vi "KI6221.vi"() -> ()   [LabVIEW 2019] (continued)
                            w597 = u16 2 ("f")
                            n439 = Equal?(x=w597, y=w598) -> (x = y?=w599:bool)
                            n440 = Select(t=w601, s=w599, f=w597) -> (s? t:f=w600:u16)
                            n441 = case shown="2" w600 {
                              tunnel: [FALSE ("VALID SETUP") TRUE ("VALID SETUP")] -> w605
                              tunnel: [TRUE ("VALID SETUP") FALSE ("VALID SETUP")] -> w604
                              frame 1, Default {
                              }
                              frame 2 {
                              }
                            }
                          }
                          frame 4 {
                            n442 = property on="GPIB 6220 label" class="Str"() -> ("Visible"=w637:bool)  [unwired: 2 in, 2 out]
                            n443 = case shown="True" w637 {
                              frame False {
                              }
                              frame True {
                                n444 = local write "Select the interface for the 6220/6221:"(2 ("Numeric 2")) -> ()
                              }
                            }
                            n445 = case shown="2, Default" w642 {
                              tunnel: [FALSE ("VALID SETUP") TRUE ("VALID SETUP")] -> w641
                              tunnel: [TRUE ("VALID SETUP") FALSE ("VALID SETUP")] -> w640
                              frame 1 {
                              }
                              frame 2, Default {
                              }
                            }
                          }
                          frame 5 {
                            n446 = local read "Verify instruments"() -> (w673:bool)
                            n447 = case shown="True" w673 {
                              tunnel: [0 2] -> w675
                              frame False {
                              }
                              frame True {
                              }
                            }
                            n448 = case shown="2, Default" w677 {
                              tunnel: [FALSE ("VALID SETUP") TRUE ("VALID SETUP")] -> w678
                              tunnel: [TRUE ("VALID SETUP") FALSE ("VALID SETUP")] -> w676
                              frame 1 {
                              }
                              frame 2, Default {
                              }
                            }
                          }
                          frame 6 {
                            n449 = local read "6220 Connect"() -> (w712:u16)
                            n450 = Equal To 0?(x=w712) -> (x = 0?=w715:bool)
                            n451 = Select(t=i16 2, s=w715, f=0 ("Numeric 2")) -> (s? t:f=w711:i32)
                            n452 = case shown="2, Default" w718 {
                              tunnel: [FALSE ("VALID SETUP") TRUE ("VALID SETUP")] -> w717
                              tunnel: [TRUE ("VALID SETUP") FALSE ("VALID SETUP")] -> w716
                              frame 1 {
                              }
                              frame 2, Default {
                              }
                            }
                          }
                          frame 7 {
                            n453 = case shown="8" w745 {
                              tunnel: [FALSE ("VALID SETUP") TRUE ("VALID SETUP")] -> w744
                              frame 0, Default {
                              }
                              frame 8 {
                              }
                            }
                            n454 = case shown="2, Default" w753 {
                              tunnel: [FALSE ("VALID SETUP") TRUE ("VALID SETUP")] -> w752
                              tunnel: [TRUE ("VALID SETUP") FALSE ("VALID SETUP")] -> w751
                              frame 1 {
                              }
                              frame 2, Default {
                              }
                            }
                          }
                          frame 8 {
                            n455 = case shown="1, 2, Default" w782 {
                              tunnel: [FALSE ("VALID SETUP") TRUE ("VALID SETUP")] -> w783
                              frame 3 {
                              }
                              frame 1, 2, Default {
                              }
                            }
                            n456 = case shown="9" w781 {
                              tunnel: [FALSE ("VALID SETUP") TRUE ("VALID SETUP")] -> w786
                              frame 0, Default {
                              }
                              frame 9 {
                              }
                            }
                            n457 = case shown="2, Default" w791 {
                              tunnel: [FALSE ("VALID SETUP") TRUE ("VALID SETUP")] -> w790
                              tunnel: [TRUE ("VALID SETUP") FALSE ("VALID SETUP")] -> w789
                              frame 1 {
                              }
                              frame 2, Default {
                              }
                            }
                          }
                          frame 9 {
                            n458 = case shown="2, Default" w829 {
                              tunnel: [FALSE ("VALID SETUP") TRUE ("VALID SETUP")] -> w828
                              tunnel: [TRUE ("VALID SETUP") FALSE ("VALID SETUP")] -> w827
                              frame 1 {
                              }
                              frame 2, Default {
                              }
                            }
                          }
                        }
                        n459 = property on="Select the current source model number:" class="Ring (strict)"("Visible"=w425, "Disabled"=w445) -> ()  [unwired: 2 in, 2 out]
                        n460 = property on="Select Network Card number:\n(default to zero)" class="DigNum (strict)"("Visible"=w439, "Disabled"=w438) -> ()  [unwired: 2 in, 2 out]
                        n461 = property on="Select the interface for the 6220/6221:" class="Ring (strict)"("Visible"=w442, "Disabled"=w441) -> ()  [unwired: 2 in, 2 out]
                        n462 = property on="Select GPIB Board number:\n(default to zero)" class="DigNum (strict)"("Visible"=w417, "Disabled"=w436) -> ()  [unwired: 2 in, 2 out]
                        n463 = property on="CANCEL" class="Bool"("Visible"=w420) -> ()  [unwired: 2 in, 2 out]
                        n464 = property on="Select the nanovoltmeter model number:" class="Ring (strict)"("Visible"=w444, "Disabled"=w443) -> ()  [unwired: 2 in, 2 out]
                        n465 = property on="Power:" class="Ring (strict)"("Visible"=w418, "Disabled"=w437) -> ()  [unwired: 2 in, 2 out]
                        n466 = property on="Select GPIB Address number \nof the current source:" class="DigNum (strict)"("Visible"=w416, "Disabled"=w440) -> ()  [unwired: 2 in, 2 out]
                        n467 = property on="NEXT" class="Bool"("Disabled"=w398) -> ()  [unwired: 2 in, 2 out]
                        n468 = Equal To 0?(x=w398) -> (x = 0?=w396:bool)
                        n469 = Not(x=w394) -> (.not. x?=w395:bool)
                        n470 = And(x=w396, y=w395) -> (x .and. y?=w397:bool)
                        n471 = case shown="True" w397 {
                          frame False {
                          }
                          frame True {
                            n472 = property on="NEXT" class="Bool"("Key Focus"=TRUE) -> ()  [unwired: 2 in, 2 out]
                          }
                        }
                        n473 = property on="instrument status" class="Str"("Visible"=w418) -> ()  [unwired: 2 in, 2 out]
                        n474 = property on="Input instrument IP Address:" class="DigNum (strict)"("Visible"=w435, "Disabled"=w434) -> ()  [unwired: 2 in, 2 out]
                        n475 = property on=".  IP#3" class="DigNum (strict)"("Visible"=w431, "Disabled"=w430) -> ()  [unwired: 2 in, 2 out]
                        n476 = property on=".  IP#2" class="DigNum (strict)"("Visible"=w433, "Disabled"=w432) -> ()  [unwired: 2 in, 2 out]
                        n477 = property on=".  IP#4" class="DigNum (strict)"("Visible"=w429, "Disabled"=w428) -> ()  [unwired: 2 in, 2 out]
                        n478 = property on="LOW to EARTH 2" class="Ring (strict)"("Visible"=w403, "Disabled"=w413) -> ()  [unwired: 2 in, 2 out]
                        n479 = property on="6220 Connect" class="Ring (strict)"("Visible"=w422, "Disabled"=w426) -> ()  [unwired: 2 in, 2 out]
                        n480 = property on="HI IMP devices?" class="Ring (strict)"("Visible"=w423, "Disabled"=w427) -> ()  [unwired: 2 in, 2 out]
                        n481 = case shown="True" w394 {
                          frame False {
                          }
                          frame True {
                            n482 = property on="OK" class="Bool (strict)"("Key Focus"=TRUE) -> ()  [unwired: 2 in, 2 out]
                          }
                        }
                        n483 = case shown="3" w401 {
                          tunnel: [TRUE FALSE] -> w400
                          frame 3 {
                          }
                          frame 1, 2, Default {
                          }
                        }
                        n484 = And(x=w400, y=w403) -> (x .and. y?=w402:bool)
                        n485 = property on="OK" class="Bool (strict)"("Visible"=w394) -> ()  [unwired: 2 in, 2 out]
                        n486 = property on="CAP IN" class="Ring (strict)"("Visible"=w402, "Disabled"=w404) -> ()  [unwired: 2 in, 2 out]
                        n487 = case shown="True" w407 {
                          tunnel: w412 -> [_ w462]
                          tunnel: w401 -> [_ w461]
                          tunnel: w411 -> [_ w460]
                          tunnel: w410 -> [_ w459]
                          tunnel: w409 -> [_ w458]
                          tunnel: w408 -> [_ w457]
                          tunnel: w406 -> [_ w451]
                          frame False {
                          }
                          frame True {
                            n488 = call "DecideWindow.vi"("Default Path"=w462, "NanoVoltmeter"=w461, "INDEX"=w451, "SOURCE 4"=w460, "MEASURE 4"=w458, "FLOAT 4"=w457, "CAP OUT 4"=w459, "wizard?"=1) -> ("SOURCE"=w455:i32, "MEASURE"=w454:i32, "FLOAT"=w453:i32, "CAP OUT"=w452:i32, "INDEX OUT"=w450:i32)  [unwired: 3 in]
                            n489 = local write "NEXT FLAG"(w450) -> ()
                            n490 = local write "LOW to EARTH 2"(w453) -> ()
                            n491 = local write "HI IMP devices?"(w454) -> ()
                            n492 = local write "6220 Connect"(w455) -> ()
                            n493 = local write "CAP IN"(w452) -> ()
                          }
                        }
                        n494 = property on="Main intro bar" class="Pict"("Visible"=w422) -> ()  [unwired: 2 in, 2 out]
                        n495 = property on="DUT connect HELP" class="Bool"("Visible"=w405) -> ()  [unwired: 2 in, 2 out]
                        n496 = property on="Src Connect HELP" class="Bool"("Visible"=w405) -> ()  [unwired: 2 in, 2 out]
                        n497 = property on="Lo earth HELP" class="Bool"("Visible"=w405) -> ()  [unwired: 2 in, 2 out]
                        n498 = property on="nVm C HELP" class="Bool"("Visible"=w405) -> ()  [unwired: 2 in, 2 out]
                      }
                    }
                  }
                  frame 1 {
                    w877 = TRUE ("Visible")
                    w885 = u8 0 ("Disabled")
                    # "PRESENT"
                    n499 = property on="Src Connect HELP" class="Bool"("Visible"=w877) -> ()  [unwired: 2 in, 2 out]
                    n500 = Equal?(x="Select the current source model number:", y=u16 2) -> (x = y?=w883:bool)
                    n501 = property on="DUT connect HELP" class="Bool"("Visible"=w877) -> ()  [unwired: 2 in, 2 out]
                    n502 = Not(x=w883) -> (.not. x?=w879:bool)
                    n503 = property on="Select the interface for the 6220/6221:" class="Ring (strict)"("Visible"=w883) -> ()  [unwired: 2 in, 2 out]
                    n504 = property on="GPIB 6220 label" class="Str"("Visible"=w879) -> ()  [unwired: 2 in, 2 out]
                    n505 = Equal?(x="Select the current source model number:", y=u16 1) -> (x = y?=w872:bool)
                    n506 = Select(t=u16 2, s=w872, f="Select the interface for the 6220/6221:") -> (s? t:f=w870:u16)
                    n507 = property on="Lo earth HELP" class="Bool"("Visible"=w877) -> ()  [unwired: 2 in, 2 out]
                    n508 = Equal?(x=w870, y=u16 2) -> (x = y?=w881:bool)
                    n509 = local write "Select the interface for the 6220/6221:"(w870) -> ()
                    n510 = Or(x=w881, y=w879) -> (x .or. y?=w878:bool)
                    n511 = Not(x=w878) -> (.not. x?=w880:bool)
                    n512 = property on="Select GPIB Address number \nof the current source:" class="DigNum (strict)"("Visible"=w878, "Disabled"=w885) -> ()  [unwired: 2 in, 2 out]
                    n513 = property on="Select GPIB Board number:\n(default to zero)" class="DigNum (strict)"("Visible"=w878, "Disabled"=w885) -> ()  [unwired: 2 in, 2 out]
                    n514 = property on=".  IP#4" class="DigNum (strict)"("Visible"=w880, "Disabled"=w885) -> ()  [unwired: 2 in, 2 out]
                    n515 = property on="Select Network Card number:\n(default to zero)" class="DigNum (strict)"("Visible"=w880, "Disabled"=w885) -> ()  [unwired: 2 in, 2 out]
                    n516 = property on="Input instrument IP Address:" class="DigNum (strict)"("Visible"=w880, "Disabled"=w885) -> ()  [unwired: 2 in, 2 out]
                    n517 = property on=".  IP#2" class="DigNum (strict)"("Visible"=w880, "Disabled"=w885) -> ()  [unwired: 2 in, 2 out]
                    n518 = property on=".  IP#3" class="DigNum (strict)"("Visible"=w880, "Disabled"=w885) -> ()  [unwired: 2 in, 2 out]
                    n519 = case shown="1, 2, Default" w876 {
                      tunnel: [TRUE FALSE] -> w875
                      frame 3 {
                      }
                      frame 1, 2, Default {
                      }
                    }
                    n520 = property on="CAP IN" class="Ring (strict)"("Visible"=w875) -> ()  [unwired: 2 in, 2 out]
                    n521 = property on="nVm C HELP" class="Bool"("Visible"=w875) -> ()  [unwired: 2 in, 2 out]
                  }
                }
                n522 = case shown="True" "nVm C HELP" {
                  tunnel: w293 -> [_ w373]
                  tunnel: "HI IMP devices?" -> [_ w372]
                  tunnel: w292 -> [_ w370]
                  tunnel: w298 -> [_ w369]
                  tunnel: "LOW to EARTH 2" -> [_ w368]
                  tunnel: "CAP IN" -> [_ w363]
                  frame False {
                  }
                  frame True {
                    n523 = call "DecideWindow.vi"("Default Path"=w369, "NanoVoltmeter"=w370, "INDEX"=3, "SOURCE 4"=w373, "MEASURE 4"=w372, "FLOAT 4"=w368, "CAP OUT 4"=w363, "wizard?"=0) -> ("SOURCE"=w367:i32, "MEASURE"=w366:i32, "FLOAT"=w365:i32, "CAP OUT"=w364:i32)  [unwired: 3 in, 1 out]
                    n524 = local write "LOW to EARTH 2"(w365) -> ()
                    n525 = local write "6220 Connect"(w367) -> ()
                    n526 = local write "HI IMP devices?"(w366) -> ()
                    n527 = local write "CAP IN"(w364) -> ()
                  }
                }
                n528 = case shown="True" "Src Connect HELP" {
                  tunnel: "CAP IN" -> [_ w360]
                  tunnel: "LOW to EARTH 2" -> [_ w359]
                  tunnel: w292 -> [_ w358]
                  tunnel: "HI IMP devices?" -> [_ w357]
                  tunnel: w293 -> [_ w356]
                  tunnel: w298 -> [_ w355]
                  frame False {
                  }
                  frame True {
                    n529 = call "DecideWindow.vi"("Default Path"=w355, "NanoVoltmeter"=w358, "INDEX"=0, "SOURCE 4"=w356, "MEASURE 4"=w357, "FLOAT 4"=w359, "CAP OUT 4"=w360, "wizard?"=0) -> ("SOURCE"=w353:i32, "MEASURE"=w352:i32, "FLOAT"=w351:i32, "CAP OUT"=w354:i32)  [unwired: 3 in, 1 out]
                    n530 = local write "LOW to EARTH 2"(w351) -> ()
                    n531 = local write "HI IMP devices?"(w352) -> ()
                    n532 = local write "6220 Connect"(w353) -> ()
                    n533 = local write "CAP IN"(w354) -> ()
                  }
                }
                n534 = case shown="True" "DUT connect HELP" {
                  tunnel: "CAP IN" -> [_ w348]
                  tunnel: "LOW to EARTH 2" -> [_ w347]
                  tunnel: w292 -> [_ w346]
                  tunnel: "HI IMP devices?" -> [_ w345]
                  tunnel: w293 -> [_ w344]
                  tunnel: w298 -> [_ w343]
                  frame False {
                  }
                  frame True {
                    n535 = call "DecideWindow.vi"("Default Path"=w343, "NanoVoltmeter"=w346, "INDEX"=1, "SOURCE 4"=w344, "MEASURE 4"=w345, "FLOAT 4"=w347, "CAP OUT 4"=w348, "wizard?"=0) -> ("SOURCE"=w342:i32, "MEASURE"=w341:i32, "FLOAT"=w340:i32, "CAP OUT"=w339:i32)  [unwired: 3 in, 1 out]
                    n536 = local write "LOW to EARTH 2"(w340) -> ()
                    n537 = local write "HI IMP devices?"(w341) -> ()
                    n538 = local write "6220 Connect"(w342) -> ()
                    n539 = local write "CAP IN"(w339) -> ()
                  }
                }
                n540 = case shown="True" "Lo earth HELP" {
                  tunnel: "CAP IN" -> [_ w336]
                  tunnel: "LOW to EARTH 2" -> [_ w335]
                  tunnel: w292 -> [_ w334]
                  tunnel: "HI IMP devices?" -> [_ w333]
                  tunnel: w293 -> [_ w332]
                  tunnel: w298 -> [_ w331]
                  frame False {
                  }
                  frame True {
                    n541 = call "DecideWindow.vi"("Default Path"=w331, "NanoVoltmeter"=w334, "INDEX"=2, "SOURCE 4"=w332, "MEASURE 4"=w333, "FLOAT 4"=w335, "CAP OUT 4"=w336, "wizard?"=0) -> ("SOURCE"=w327:i32, "MEASURE"=w328:i32, "FLOAT"=w329:i32, "CAP OUT"=w330:i32)  [unwired: 3 in, 1 out]
                    n542 = local write "LOW to EARTH 2"(w329) -> ()
                    n543 = local write "HI IMP devices?"(w328) -> ()
                    n544 = local write "6220 Connect"(w327) -> ()
                    n545 = local write "CAP IN"(w330) -> ()
                  }
                }
                n546 = case shown="True" "Case Constant\n(See Context Help) 3" {
                  tunnel: w292 -> [_ w323]
                  frame False {
                  }
                  frame True {
                    n547 = case shown="3" w323 {
                      tunnel: [TRUE FALSE] -> w324
                      frame 3 {
                      }
                      frame 1, 2, Default {
                      }
                    }
                    n548 = property on="nVm C HELP" class="Bool"("Visible"=w324) -> ()  [unwired: 2 in, 2 out]
                    n549 = property on="CAP IN" class="Ring (strict)"("Visible"=w324) -> ()  [unwired: 2 in, 2 out]
                  }
                }
                n550 = call "Measure Connect HELP"("Enable"=w303) -> ()  [unwired: 9 in, 2 out]
                n551 = call "Low to Earth HELP"("Enable"=w303) -> ()  [unwired: 9 in, 2 out]
                n552 = call "Source Connect HELP"("Enable"=w303) -> ()  [unwired: 9 in, 2 out]
              }
              frame "CONN GUIDE" {
                w1092 = u8 0 ("Disabled")
                # "How Do I Decide Links"
                # "BUTTONS INVISIBLE IN THIS VERSION OF THE PANEL."
                # "Global Buttons"
                # "PREVIOUS & START OVER BUTTON CONTROLS"
                # "GUIDE BUTTON CONTROLS"
                n553 = Not Equal?(x="4 step TABS", y="4 step TABS LAST") -> (x != y?=w1096:bool)
                n554 = case shown="True" "END OF GUIDE" {
                  frame False {
                  }
                  frame True {
                    n555 = local write "4 step TABS"(T3."step 4" ("4 step TABS")) -> ()
                  }
                }
                n556 = case shown="True" "start of guide" {
                  frame False {
                  }
                  frame True {
                    n557 = local write "4 step TABS"(T3."step 1" ("4 step TABS")) -> ()
                  }
                }
                n558 = case shown="True" "Previous" {
                  tunnel: "4 step TABS" -> [_ w1211]
                  frame False {
                  }
                  frame True {
                    n559 = Decrement(x=w1211) -> (x-1=w1210:T3)
                    n560 = local write "4 step TABS"(w1210) -> ()
                  }
                }
                n561 = property on="Main Tabs" class="TabCtl (strict)"("Page Selector Visible"=TRUE) -> ()  [unwired: 2 in, 2 out]
                n562 = case shown="True" "NEXT GUIDE" {
                  tunnel: "4 step TABS" -> [_ w1209]
                  frame False {
                  }
                  frame True {
                    n563 = Increment(x=w1209) -> (x+1=w1208:T3)
                    n564 = local write "4 step TABS"(w1208) -> ()
                  }
                }
                n565 = case shown="True" w1096 {
                  tunnel: "4 step TABS" -> [_ w1191]
                  frame False {
                  }
                  frame True {
                    n566 = case shown="\"step 4\"" w1191 {
                      tunnel: [u8 2 ("Disabled") w1198 u8 0 ("Disabled") w1203 w1205] -> w1193
                      tunnel: [u8 0 ("Disabled") w1198 u8 2 ("Disabled") w1203 w1205] -> w1192
                      tunnel: [FALSE FALSE TRUE FALSE FALSE] -> w1190
                      frame "step 1", Default {
                      }
                      frame "step 3" {
                        w1198 = u8 0 ("Disabled")
                      }
                      frame "step 4" {
                      }
                      frame "final" {
                        w1203 = u8 0 ("Disabled")
                      }
                      frame "step 2" {
                        w1205 = u8 0 ("Disabled")
                      }
                    }
                    n567 = local write "4 step TABS LAST"(w1191) -> ()
                    n568 = property on="start of guide" class="Bool"("Disabled"=w1193) -> ()  [unwired: 2 in, 2 out]
                    n569 = property on="Previous" class="Bool"("Disabled"=w1193) -> ()  [unwired: 2 in, 2 out]
                    n570 = property on="END OF GUIDE" class="Bool"("Disabled"=w1192) -> ()  [unwired: 2 in, 2 out]
                    n571 = property on="NEXT GUIDE" class="Bool"("Disabled"=w1192) -> ()  [unwired: 2 in, 2 out]
                    n572 = property on="Nearby AC voltages" class="Bool (strict)"("Visible"=w1190) -> ()  [unwired: 2 in, 2 out]
                    n573 = property on="AC HELP" class="Bool"("Visible"=w1190) -> ()  [unwired: 2 in, 2 out]
                    n574 = property on="HAZARD HELP" class="Bool"("Visible"=w1190) -> ()  [unwired: 2 in, 2 out]
                    n575 = property on="H,L,G Haz volt" class="Bool (strict)"("Visible"=w1190) -> ()  [unwired: 2 in, 2 out]
                  }
                }
                n576 = property on="EXIT 2" class="Bool (strict)"("Disabled"=w1092) -> ()  [unwired: 2 in, 2 out]
                n577 = property on="SAVE 2" class="Bool"("Disabled"=w1092) -> ()  [unwired: 2 in, 2 out]
                n578 = case shown="True" "setup wizard" {
                  frame False {
                  }
                  frame True {
                    n579 = case shown="True" "CONNECT\nONLY FLAG" {
                      tunnel: [T2."CONN CONFIG" ("COMM\nTab Control") T2."STARTUP" ("COMM\nTab Control")] -> w1214
                      frame False {
                      }
                      frame True {
                      }
                    }
                    n580 = property on="COMM\nTab Control" class="TabCtl (strict)"("Value"=w1214) -> ()  [unwired: 2 in, 2 out]
                  }
                }
                n581 = case shown="True" "RETURN TO SPLASH SCREEN" {
                  frame False {
                  }
                  frame True {
                    n582 = property on="COMM\nTab Control" class="TabCtl (strict)"("Value"=T2."STARTUP" ("COMM\nTab Control")) -> ()  [unwired: 2 in, 2 out]
                  }
                }
                n583 = Not Equal?(x="Nearby AC voltages", y="Nearby AC voltages LAST") -> (x != y?=w1087:bool)
                n584 = Not Equal?(x="H,L,G Haz volt", y="H,L,G Haz volt LAST") -> (x != y?=w1086:bool)
                n585 = Not Equal?(x="CAP", y="CAP LAST") -> (x != y?=w1085:bool)
                n586 = Not Equal?(x="COMM TAB LAST", y=w1093) -> (x != y?=w1081:bool)
                n587 = Compound Arithmetic op=OR(w1081, w1087, w1086, w1085) -> (w1088:bool)
                n588 = case shown="True" w1088 {
                  tunnel: w1093 -> [_ w1166]
                  tunnel: "Nearby AC voltages" -> [_ w1116]
                  tunnel: "H,L,G Haz volt" -> [_ w1114]
                  tunnel: "CAP" -> [_ w1117]
                  tunnel: w1081 -> [_ w1113]
                  frame False {
                  }
                  frame True {
                    w1122 = ".png" ("string")
                    w1129 = "Guide" ("string")
                    # "Initialize pictures when you get to the GUIDE GUI PANEL."
                    n589 = local read "6220 Connect"() -> (w1115:u16)
                    n590 = local read "Select the interface for the 6220/6221:"() -> (w1167:u16)
                    n591 = local write "COMM TAB LAST"(w1166) -> ()
                    n592 = Decrement(x=w1115) -> (x-1=w1139:u16)
                    n593 = Number To Decimal String(number=w1139) -> (decimal integer string=w1138:string)  [unwired: 1 in]
                    n594 = local read "LOW to EARTH 2"() -> (w1168:u16)
                    n595 = Number To Decimal String(number=w1168) -> (decimal integer string=w1118:string)  [unwired: 1 in]
                    n596 = local write "CAP LAST"(w1117) -> ()
                    n597 = local read "Default path"() -> (w1130:path)
                    n598 = local read "HI IMP devices?"() -> (w1121:u16)
                    n599 = Decrement(x=w1167) -> (x-1=w1163:u16)
                    n600 = Number To Decimal String(number=w1163) -> (decimal integer string=w1128:string)  [unwired: 1 in]
                    n601 = case shown="1" w1121 {
                      tunnel: [u16 1 ("HI IMP devices?") u16 0 ("HI IMP devices?")] -> w1120
                      frame 0, Default {
                      }
                      frame 1 {
                      }
                    }
                    n602 = Number To Decimal String(number=w1120) -> (decimal integer string=w1119:string)  [unwired: 1 in]
                    n603 = Boolean To (0,1)(Boolean=w1116) -> (0, 1=w1165:i16)
                    n604 = local write "Nearby AC voltages LAST"(w1116) -> ()
                    n605 = Number To Decimal String(number=w1165) -> (decimal integer string=w1157:string)  [unwired: 1 in]
                    n606 = Number To Decimal String(number=2 ("y")) -> (decimal integer string=w1143:string)  [unwired: 1 in]
                    n607 = Number To Decimal String(number=4 ("y")) -> (decimal integer string=w1159:string)  [unwired: 1 in]
                    n608 = Number To Decimal String(number=1 ("y")) -> (decimal integer string=w1134:string)  [unwired: 1 in]
                    n609 = Concatenate Strings(w1129, w1143, w1138, w1118, w1122) -> (w1144:string)
                    n610 = Concatenate Strings(w1129, w1134, w1128, w1122) -> (w1135:string)
                    n611 = Build Path(base path=w1130, name or relative path=w1144) -> (appended path=w1146:path)
                    n612 = Build Path(base path=w1130, name or relative path=w1135) -> (appended path=w1137:path)
                    n613 = call <vilib>:"Read PNG File.vi"("path to PNG file"=w1146) -> ("error out"=w1141:errorcluster, "image data"=w1145:T13)  [unwired: 8 in, 1 out]
                    n614 = Number To Decimal String(number=3 ("y")) -> (decimal integer string=w1150:string)  [unwired: 1 in]
                    n615 = Concatenate Strings(w1129, w1150, w1119, w1122) -> (w1151:string)
                    n616 = Build Path(base path=w1130, name or relative path=w1151) -> (appended path=w1153:path)
                    n617 = call <vilib>:"Read PNG File.vi"("path to PNG file"=w1137) -> ("error out"=w1132:errorcluster, "image data"=w1136:T13)  [unwired: 8 in, 1 out]
                    n618 = call <vilib>:"Read PNG File.vi"("path to PNG file"=w1153) -> ("error out"=w1148:errorcluster, "image data"=w1152:T13)  [unwired: 8 in, 1 out]
                    n619 = call <vilib>:"Draw Flattened Pixmap.vi"("image data"=w1145) -> ("new picture"=w1140:picture)  [unwired: 8 in]
                    n620 = case shown="2, Default" w1115 {
                      tunnel: [2 ("y") 0 ("y")] -> w1112
                      tunnel: [TRUE ("H,L,G Haz volt") w1174] -> w1111
                      tunnel: w1114 -> [_ w1174]
                      frame 2, Default {
                      }
                      frame 1 {
                      }
                    }
                    n621 = Boolean To (0,1)(Boolean=w1111) -> (0, 1=w1164:i16)
                    n622 = Number To Decimal String(number=w1164) -> (decimal integer string=w1156:string)  [unwired: 1 in]
                    n623 = Concatenate Strings(w1129, w1159, w1138, w1119, w1118, w1157, w1156, w1122) -> (w1160:string)
                    n624 = Build Path(base path=w1130, name or relative path=w1160) -> (appended path=w1162:path)
                    n625 = call <vilib>:"Read PNG File.vi"("path to PNG file"=w1162) -> ("error out"=w1155:errorcluster, "image data"=w1161:T13)  [unwired: 8 in, 1 out]
                    n626 = call <vilib>:"Draw Flattened Pixmap.vi"("image data"=w1161) -> ("new picture"=w1154:picture)  [unwired: 8 in]
                    n627 = case shown="No Error" w1155 {
                      tunnel: w1154 -> [w1188 _]
                      tunnel: [FALSE TRUE] -> w1126
                      frame No Error {
                        n628 = local write "step 4 pic"(w1188) -> ()
                      }
                      frame Error {
                      }
                    }
                    n629 = call <vilib>:"Draw Flattened Pixmap.vi"("image data"=w1136) -> ("new picture"=w1131:picture)  [unwired: 8 in]
                    n630 = call <vilib>:"Draw Flattened Pixmap.vi"("image data"=w1152) -> ("new picture"=w1147:picture)  [unwired: 8 in]
                    n631 = case shown="No Error" w1141 {
                      tunnel: w1140 -> [w1182 _]
                      tunnel: [FALSE TRUE] -> w1124
                      frame No Error {
                        n632 = local write "step 2 pic"(w1182) -> ()
                      }
                      frame Error {
                      }
                    }
                    n633 = case shown="No Error" w1132 {
                      tunnel: w1131 -> [w1179 _]
                      tunnel: [FALSE TRUE] -> w1123
                      frame No Error {
                        n634 = local write "step 1 pic"(w1179) -> ()
                      }
                      frame Error {
                      }
                    }
                    n635 = case shown="No Error" w1148 {
                      tunnel: w1147 -> [w1185 _]
                      tunnel: [FALSE TRUE] -> w1125
                      frame No Error {
                        n636 = local write "step 3 pic"(w1185) -> ()
                      }
                      frame Error {
                      }
                    }
                    n637 = property on="H,L,G Haz volt" class="Bool (strict)"("Value"=w1111, "Disabled"=w1112) -> ()  [unwired: 2 in, 2 out]
                    n638 = case shown="True" w1113 {
                      frame False {
                      }
                      frame True {
                        n639 = local write "4 step TABS"(T3."step 1" ("4 step TABS")) -> ()
                        n640 = property on="NEXT GUIDE" class="Bool"("Disabled"=u8 0) -> ()  [unwired: 2 in, 2 out]
                        n641 = property on="Previous" class="Bool"("Disabled"=u8 2) -> ()  [unwired: 2 in, 2 out]
                      }
                    }
                    n642 = local write "H,L,G Haz volt LAST"(w1111) -> ()
                    n643 = property on="HAZARD HELP" class="Bool"("Disabled"=w1112) -> ()  [unwired: 2 in, 2 out]
                    n644 = Compound Arithmetic op=OR(w1126, w1125, w1124, w1123) -> (w1127:bool)
                    n645 = call "Images not found"("Enable"=w1127) -> ()  [unwired: 9 in, 2 out]
                  }
                }
                n646 = local read "Default path"() -> (w1078:path)
                n647 = case shown="True" "HAZARD HELP" {
                  tunnel: w1078 -> [_ w1108]
                  frame False {
                  }
                  frame True {
                    n648 = call "DecideWindow.vi"("Default Path"=w1108, "INDEX"=5, "wizard?"=0) -> ()  [unwired: 8 in, 5 out]
                  }
                }
                n649 = case shown="True" "AC HELP" {
                  tunnel: w1078 -> [_ w1105]
                  frame False {
                  }
                  frame True {
                    n650 = call "DecideWindow.vi"("Default Path"=w1105, "INDEX"=6, "wizard?"=0) -> ()  [unwired: 8 in, 5 out]
                  }
                }
              }
              frame "STEP CONFIG" {
                w1218 = u8 2 ("Disabled")
                # "Step setup CANCEL. Returns all VARS to previous values."
                # "This vi updates the VARS for the step source. Used when OK is \nclicked."
                # "Controls/Indicators referenced, not used."
                # "This enables the OK button once a name is entered."
                # "Turns off TABS MUST HIT OK or CANCEL to CONTINUE."
                n651 = case shown="True" "step setup OK" {
                  frame False {
                  }
                  frame True {
                    n652 = control-ref of="STEP EDIT VAR"() -> (w1230:refnum<vi>)
                    n653 = control-ref of="GPIB Address:"() -> (w1238:refnum<vi>)
                    n654 = control-ref of="DELAY in mS"() -> (w1232:refnum<vi>)
                    n655 = control-ref of="GO TO LEVEL:                *NOTE - MUST include <LEVEL>"() -> (w1239:refnum<vi>)
                    n656 = control-ref of="INSTRUMENT NAME:"() -> (w1237:refnum<vi>)
                    n657 = control-ref of="VERIFY:"() -> (w1236:refnum<vi>)
                    n658 = control-ref of="RESPONSE STRING:"() -> (w1235:refnum<vi>)
                    n659 = control-ref of="CONFIGURE:"() -> (w1234:refnum<vi>)
                    n660 = control-ref of="DEACTIVATE:"() -> (w1233:refnum<vi>)
                    n661 = control-ref of="MASTER DRIVER Array"() -> (w1231:refnum<vi>)
                    n662 = control-ref of="Default path"() -> (w1241:refnum<vi>)
                    n663 = control-ref of="Select step source:"() -> (w1240:refnum<vi>)
                    n664 = control-ref of="Advanced Operation Tab"() -> (w1229:refnum<vi>)
                    n665 = control-ref of="Main Tabs"() -> (w1228:refnum<vi>)
                    n666 = call "StepSrcUpdate.vi"("Big Tabs"=w1228, "Delay in ms"=w1232, "Step Edit Var"=w1230, "Main Window Tabs"=w1229, "RESPONSE STRING"=w1235, "Default Path"=w1241, "DEACTIVATE"=w1233, "Step Source"=w1240, "VERIFY"=w1236, "GPIB ADDRESS"=w1238, "CONMFIGURE"=w1234, "INSTRUMENT NAME"=w1237, "GO TO LEVEL"=w1239, "Master Array"=w1231) -> ("error out 33"=→"error out 33":errorcluster)  [unwired: 1 in]
                  }
                }
                n667 = property on="Main Tabs" class="TabCtl (strict)"("Page Selector Visible"=FALSE) -> ()  [unwired: 2 in, 2 out]
                n668 = property on="SAVE 2" class="Bool"("Disabled"=w1218) -> ()  [unwired: 2 in, 2 out]
                n669 = property on="EXIT 2" class="Bool (strict)"("Disabled"=w1218) -> ()  [unwired: 2 in, 2 out]
                n670 = String Length(string="INSTRUMENT NAME:") -> (length=w1225:i32)
                n671 = Equal?(x=w1225, y=u8 0 ("Disabled")) -> (x = y?=w1224:bool)
                n672 = Boolean To (0,1)(Boolean=w1224) -> (0, 1=w1223:i16)
                n673 = case shown="True" "step setup CANCEL" {
                  frame False {
                  }
                  frame True {
                    n674 = property on="STEP EDIT VAR" class="Bool (strict)"() -> ("Value"=w1247:bool)  [unwired: 2 in, 2 out]
                    n675 = case shown="False" w1247 {
                      tunnel: [0 w1249] -> w1246
                      frame False {
                      }
                      frame True {
                        n676 = property on="Select step source:" class="Ring (strict)"() -> ("Value"=w1249:u16)  [unwired: 2 in, 2 out]
                      }
                    }
                    n677 = local write "Advanced Operation Tab"(T4."Differential Conductance Measurements" ("Main Window Tabs")) -> ()
                    n678 = local write "COMM\nTab Control"(T2."STARTUP" ("COMM\nTab Control")) -> ()
                    n679 = local write "Main Tabs"(T1."Advanced Operation" ("Big Tabs")) -> ()
                    n680 = property on="Select step source:" class="Ring (strict)"("Value"=w1246) -> ()  [unwired: 2 in, 2 out]
                  }
                }
                n681 = Multiply(x=i16 2, y=w1223) -> (x*y=w1222:i16)
                n682 = property on="step setup OK" class="Bool"("Disabled"=w1222) -> ()  [unwired: 2 in, 2 out]
              }
            }
          }
          frame "Basic Operation" {
            n683 = local read "DEMO MODE"() -> (w1250:bool)
            n684 = case shown="\"DC Sweep\"" "Basic Source" {
              selector: "Basic Source" -> [w1259 w1349 w1710]
              tunnel: w1250 -> [w1256 w1322 w1702]
              frame "DC Source", Default {
                n685 = Not Equal?(x="Current Source \nVoltage Compliance (V)", y="Current Source \nVoltage Compliance (V) LAST") -> (x != y?=w1266:bool)
                n686 = Not Equal?(x="Source Level (Amps)", y="Source Level (Amps) LAST") -> (x != y?=w1267:bool)
                n687 = Not Equal?(x="Activate Output", y="Activate Output LAST") -> (x != y?=w1265:bool)
                n688 = Compound Arithmetic op=OR(w1267, w1266, w1265) -> (w1264:bool)
                n689 = And(x="init", y="TAKE CONTROL") -> (x .and. y?=w1253:bool)
                n690 = Not(x=w1256) -> (.not. x?=w1257:bool)
                n691 = Compound Arithmetic op=AND(w1257, w1264, "TAKE CONTROL") -> (w1258:bool)
                n692 = Or(x=w1253, y=w1258) -> (x .or. y?=w1255:bool)
                n693 = case shown="True" w1255 {
                  tunnel: "Source Level (Amps)" -> [_ w1284]
                  tunnel: "Current Source \nVoltage Compliance (V)" -> [_ w1283]
                  tunnel: "Activate Output" -> [_ w1282]
                  tunnel: "Source TABS LAST" -> [_ w1279]
                  tunnel: w1259 -> [_ w1278]
                  frame False {
                  }
                  frame True {
                    n694 = local write "Current Source \nVoltage Compliance (V) LAST"(w1283) -> ()
                    n695 = local write "Source Level (Amps) LAST"(w1284) -> ()
                    n696 = local write "Activate Output LAST"(w1282) -> ()
                    n697 = local read "Setup String"() -> (w1275:string)
                    n698 = local read "6220 VISA"() -> (w1285:refnum<visa-resource-name>)
                    n699 = local read "GPIB Array"() -> (w1277:string[])
                    n700 = Insert Into Array(array=string[] [], new element=w1275) -> (w1273:string[])  [unwired: 1 in]
                    n701 = call "VisaVarReplace.vi"("Replace Array"=w1273, "Search Array"=string[] ["<SETUPSTRING>"], "GPIB Array"=w1277) -> ("GPIB Array OUT"=w1276:string[])
                    n702 = call "VISAreadWrite.vi"("GPIB INDEX Array"=i32[] [37], "GPIB ARRAY"=w1276, "VISA REFERENCE"=w1285) -> ("error out 15"=w1281:errorcluster, "Read Buffer Array"=w1289:string[])  [unwired: 1 in]
                    n703 = Index Array(array=w1289, index=1) -> (element=w1291:string)
                    n704 = Match Pattern(string=w1291, regular expression="MODEL 622") -> (offset past match=w1288:i32)  [unwired: 1 in, 3 out]
                    n705 = local write "init"(FALSE ("init")) -> ()
                    n706 = Not Equal?(x=w1288, y=-1) -> (x != y?=w1286:bool)
                    n707 = case shown="True" w1286 {
                      tunnel: w1285 -> [_ w1313]
                      tunnel: w1277 -> [_ w1312]
                      tunnel: w1284 -> [_ w1303]
                      tunnel: w1283 -> [_ w1302]
                      tunnel: w1282 -> [_ w1305]
                      tunnel: w1281 -> [w1296 w1315]
                      tunnel: [w1295 w1314] -> w1280
                      tunnel: w1279 -> [_ w1299]
                      tunnel: w1278 -> [_ w1297]
                      frame False {
                        # "no instr"
                        n708 = call "No 6220/6221 responding"("error in (no error)"=w1296) -> ("error out"=w1295:errorcluster)  [unwired: 9 in, 1 out]
                        n709 = local write "TAKE CONTROL"(FALSE ("TAKE CONTROL")) -> ()
                      }
                      frame True {
                        # "found"
                        n710 = Number To Exponential String(number=w1303) -> (E-format string=w1300:string)  [unwired: 3 in]
                        n711 = case shown="True" w1305 {
                          tunnel: ["off" "on"] -> w1304
                          frame False {
                          }
                          frame True {
                          }
                        }
                        n712 = Number To Exponential String(number=w1302) -> (E-format string=w1301:string)  [unwired: 3 in]
                        n713 = Insert Into Array(array=string[] [], new element=w1300) -> (w1309:string[])  [unwired: 1 in]
                        n714 = Insert Into Array(array=w1309, new element=w1301) -> (w1308:string[])  [unwired: 1 in]
                        n715 = Insert Into Array(array=w1308, new element=w1304) -> (w1307:string[])  [unwired: 1 in]
                        n716 = call "VisaVarReplace.vi"("Replace Array"=w1307, "Search Array"=string[] ["<SOURCE>", "<COMPLIANCE>", "<OUTPUT>"], "GPIB Array"=w1312) -> ("GPIB Array OUT"=w1316:string[])
                        n717 = Not Equal?(x=w1297, y=w1299) -> (x != y?=w1298:bool)
                        n718 = case shown="True" w1298 {
                          tunnel: [i32[] [29] ("GPIB INDEX Array") i32[] [29] ("GPIB INDEX Array")] -> w1311
                          tunnel: w1297 -> [_ w1319]
                          frame False {
                          }
                          frame True {
                            n719 = local write "Source TABS LAST"(w1319) -> ()
                          }
                        }
                        n720 = call "VISAreadWrite.vi"("error in (no error)"=w1315, "GPIB INDEX Array"=w1311, "GPIB ARRAY"=w1316, "VISA REFERENCE"=w1313) -> ("error out 15"=w1314:errorcluster)  [unwired: 1 out]
                      }
                    }
                    "error" <- w1280
                  }
                }
              }
              frame "DC Sweep" {
                # "TRAC:DATA? with full buffer on ENET causes SYSTEM ERROR on 6221\nmaybe...,"
                # "SETUP STRINGS"
                n721 = local read "GPIB Array"() -> (w1328:string[])
                n722 = local read "6220 VISA"() -> (w1329:refnum<visa-resource-name>)
                n723 = Not(x=w1322) -> (.not. x?=w1325:bool)
                n724 = And(x=w1325, y="RUN SWEEP") -> (x .and. y?=w1326:bool)
                n725 = local write "Source TABS LAST"(w1349) -> ()
                n726 = case shown="True" w1326 {
                  tunnel: w1328 -> [_ w1395]
                  tunnel: w1329 -> [_ w1396]
                  tunnel: "Number of sweep points" -> [_ w1390]
                  tunnel: "Sweep Type" -> [_ w1383]
                  tunnel: "Start Current (Amps)" -> [_ w1379]
                  tunnel: "Stop Current (Amps)" -> [_ w1378]
                  tunnel: "Current Source \nVoltage Compliance (V)" -> [_ w1389]
                  tunnel: "Delay (settle time in sec)" -> [_ w1388]
                  tunnel: "Voltage Measure Range" -> [_ w1387]
                  tunnel: "Measurement Integration \n(NPLCs)" -> [_ w1386]
                  frame False {
                  }
                  frame True {
                    # "1024 max points with measure"
                    # "NOT 6221"
                    n727 = call "VISAreadWrite.vi"("GPIB INDEX Array"=i32[] [0, 12], "GPIB ARRAY"=w1395, "VISA REFERENCE"=w1396) -> ("error out 15"=→"error out 18":errorcluster, "Read Buffer Array"=w1400:string[])  [unwired: 1 in]
                    n728 = Index Array(array=w1400, index=1) -> (element=w1402:string)
                    n729 = case shown="True" "enable measure" {
                      tunnel: w1400 -> [_ w1695]
                      tunnel: [FALSE w1694] -> w1397
                      frame False {
                      }
                      frame True {
                        # "no NV"
                        n730 = Index Array(array=w1695, index=3) -> (element=w1697:string)
                        n731 = Decimal String To Number(string=w1697) -> (number=w1698:i32)  [unwired: 2 in, 1 out]
                        n732 = Equal To 0?(x=w1698) -> (x = 0?=w1694:bool)
                      }
                    }
                    n733 = Greater Or Equal?(x=w1390, y=1025) -> (x >= y?=w1393:bool)
                    n734 = Match Pattern(string=w1402, regular expression="MODEL 622") -> (offset past match=w1406:i32)  [unwired: 1 in, 3 out]
                    n735 = Equal?(x=w1406, y=-1) -> (x = y?=w1398:bool)
                    n736 = And(x=w1393, y="enable measure") -> (x .and. y?=w1391:bool)
                    n737 = Equal?(x=w1383, y=u16 1) -> (x = y?=w1377:bool)
                    n738 = Equal To 0?(x=w1379) -> (x = 0?=w1380:bool)
                    n739 = Equal To 0?(x=w1378) -> (x = 0?=w1381:bool)
                    n740 = Or(x=w1381, y=w1380) -> (x .or. y?=w1384:bool)
                    n741 = And(x=w1384, y=w1377) -> (x .and. y?=w1376:bool)
                    n742 = Compound Arithmetic op=OR(w1376, w1398, w1397, w1391, "ABORT SWEEP") -> (w1399:bool)
                    n743 = case shown="False" w1399 {
                      tunnel: w1398 -> [_ w1685]
                      tunnel: w1397 -> [_ w1684]
                      tunnel: "enable measure" -> [w1430 _]
                      tunnel: w1396 -> [w1429 _]
                      tunnel: w1395 -> [w1428 _]
                      tunnel: w1391 -> [_ w1683]
                      tunnel: w1383 -> [w1410 _]
                      tunnel: w1390 -> [w1420 _]
                      tunnel: w1379 -> [w1433 _]
                      tunnel: w1378 -> [w1422 _]
                      tunnel: w1389 -> [w1444 _]
                      tunnel: w1388 -> [w1435 _]
                      tunnel: w1387 -> [w1439 _]
                      tunnel: w1386 -> [w1436 _]
                      tunnel: w1376 -> [_ w1682]
                      frame False {
                        w1424 = FALSE ("Page Selector Visible")
                        # "good to go on config"
                        n744 = invoke on="I Sweep V Measure Data" class="Table" method="Reinit To Default"() -> ()  [unwired: 3 in, 3 out]
                        n745 = invoke on="I Sweep Graph" class="WaveformGraph (strict)" method="Reinit To Default"() -> ()  [unwired: 3 in, 3 out]
                        n746 = local read "Setup String"() -> (w1455:string)
                        n747 = case shown="False" w1430 {
                          tunnel: [i32[] [30] ("GPIB INDEX Array") i32[] [35] ("GPIB INDEX Array")] -> w1459
                          frame False {
                          }
                          frame True {
                          }
                        }
                        n748 = property on="ABORT SWEEP" class="Bool (strict)"("Disabled"=u8 0) -> ()  [unwired: 2 in, 2 out]
                        n749 = property on="RUN SWEEP" class="Bool"("Disabled"=u8 2) -> ()  [unwired: 2 in, 2 out]
                        n750 = Insert Into Array(array=string[] [], new element=w1455) -> (w1454:string[])  [unwired: 1 in]
                        n751 = Number To Decimal String(number=w1420) -> (decimal integer string=w1445:string)  [unwired: 1 in]
                        n752 = case shown="0, Default" w1410 {
                          tunnel: ["lin\n:sour:swe:rang best" ("Setup String") "log\n:sour:swe:rang auto" ("Setup String")] -> w1446
                          tunnel: w1433 -> [w1646 w1662]
                          tunnel: w1420 -> [w1644 w1666]
                          tunnel: w1422 -> [w1645 w1665]
                          tunnel: [w1640 w1663] -> w1434
                          tunnel: [TRUE w1659] -> w1423
                          frame 0, Default {
                            n753 = xnode "LIN step formula"("Start"=w1646, "Stop"=w1645, "Points"=w1644) -> ("Result"=w1643:dbl)  [unwired: 1 in, 1 out]
                            n754 = To Double Precision Float(number=w1643) -> (double precision float=w1640:dbl)
                          }
                          frame 1 {
                            n755 = Absolute Value(x=w1665) -> (abs(x)=w1660:dbl)
                            n756 = Absolute Value(x=w1662) -> (abs(x)=w1661:dbl)
                            n757 = xnode "LOG step Formula"("Start"=w1661, "Stop"=w1660, "Points"=w1666) -> ("Result"=w1664:dbl)  [unwired: 1 in, 1 out]
                            n758 = Greater Than 0?(x=w1662) -> (x > 0?=w1659:bool)
                            n759 = To Double Precision Float(number=w1664) -> (double precision float=w1663:dbl)
                          }
                        }
                        n760 = Insert Into Array(array=w1454, new element=w1446) -> (w1453:string[])  [unwired: 1 in]
                        n761 = Insert Into Array(array=w1453, new element=w1445) -> (w1452:string[])  [unwired: 1 in]
                        n762 = case shown="1" w1410 {
                          tunnel: ["BEST" "AUTO"] -> w1411
                          frame 0, Default {
                          }
                          frame 1 {
                          }
                        }
                        n763 = Number To Exponential String(number=w1422) -> (E-format string=w1442:string)  [unwired: 3 in]
                        n764 = Number To Exponential String(number=w1433) -> (E-format string=w1443:string)  [unwired: 3 in]
                        n765 = Insert Into Array(array=w1452, new element=w1443) -> (w1451:string[])  [unwired: 1 in]
                        n766 = Insert Into Array(array=w1451, new element=w1442) -> (w1450:string[])  [unwired: 1 in]
                        n767 = Multiply(x=1000.0, y=w1435) -> (x*y=w1421:dbl)
                        n768 = Number To Exponential String(number=w1444) -> (E-format string=w1441:string)  [unwired: 3 in]
                        n769 = Insert Into Array(array=w1450, new element=w1441) -> (w1449:string[])  [unwired: 1 in]
                        n770 = Number To Exponential String(number=w1435) -> (E-format string=w1440:string)  [unwired: 3 in]
                        n771 = Insert Into Array(array=w1449, new element=w1440) -> (w1448:string[])  [unwired: 1 in]
                        n772 = Multiply(x=w1420, y=16) -> (x*y=w1418:i32)
                        n773 = property on="Basic Source" class="TabCtl (strict)"("Page Selector Visible"=w1424) -> ()  [unwired: 2 in, 2 out]
                        n774 = property on="Main Tabs" class="TabCtl (strict)"("Page Selector Visible"=w1424) -> ()  [unwired: 2 in, 2 out]
                        n775 = Subtract(x=w1418, y=255) -> (x-y=w1416:i32)
                        n776 = Number To Exponential String(number=w1439) -> (E-format string=w1437:string)  [unwired: 3 in]
                        n777 = Insert Into Array(array=w1448, new element=w1437) -> (w1447:string[])  [unwired: 1 in]
                        n778 = Divide(x=w1416, y=254) -> (x/y=w1414:dbl)
                        n779 = Round Toward +Infinity(x=w1414) -> (ceil(x): smallest int >= x=w1413:dbl)
                        n780 = Number To Exponential String(number=w1436) -> (E-format string=w1438:string)  [unwired: 3 in]
                        n781 = Insert Into Array(array=w1447, new element=w1438) -> (w1408:string[])  [unwired: 1 in]
                        n782 = Insert Into Array(array=w1408, new element=w1411) -> (w1409:string[])  [unwired: 1 in]
                        n783 = call "VisaVarReplace.vi"("Replace Array"=w1409, "Search Array"=string[] ["<SETUPSTRING>", "<SPACING>", "<POINTS>", "<STARTLEVEL>", "<STOPLEVEL>", "<COMPLIANCE>", "<DELAY>", "<VOLTRANGE>", "<NPLC>", "<SWEEPRANGE>"], "GPIB Array"=w1428) -> ("GPIB Array OUT"=w1458:string[])
                        n784 = call "VISAreadWrite.vi"("GPIB INDEX Array"=w1459, "GPIB ARRAY"=w1458, "VISA REFERENCE"=w1429) -> ("error out 15"=w1427:errorcluster)  [unwired: 1 in, 1 out]
                        n785 = To Word Integer(number=w1413) -> (16bit integer=w1412:i16)
                        n786 = case shown="True" w1430 {
                          tunnel: w1429 -> [w1466 w1501]
                          tunnel: w1428 -> [w1465 w1500]
                          tunnel: w1434 -> [_ w1507]
                          tunnel: w1433 -> [_ w1506]
                          tunnel: w1427 -> [_ w1499]
                          tunnel: [TRUE TRUE] -> w1425
                          tunnel: w1410 -> [_ w1504]
                          tunnel: w1423 -> [_ w1503]
                          tunnel: w1422 -> [w1464 _]
                          tunnel: w1421 -> [w1463 _]
                          tunnel: w1412 -> [_ w1502]
                          frame False {
                            n787 = while {
                              tunnel: w1466 -> [w1470]
                              tunnel: w1465 -> [w1469]
                              tunnel: w1464 -> [w1481]
                              tunnel: w1463 -> [w1476]
                              shift-right: [w1479] -> _
                              shift-left: 1.0 -> [w1478]
                              stop <- w1480 stop-if-true
                              n788 = flat-sequence {
                                tunnel: w1476 -> [w1486]
                                tunnel: w1470 -> [w1490]
                                tunnel: w1469 -> [w1489]
                                tunnel: [w1487] -> w1468
                                frame #0 {
                                n789 = Multiply(x=2.0, y=w1486) -> (x*y=w1484:dbl)
                                n790 = Wait (ms)(milliseconds to wait=w1484) -> ()  [unwired: 1 out]
                                }
                                frame #1 {
                                n791 = call "VISAreadWrite.vi"("GPIB INDEX Array"=i32[] [46], "GPIB ARRAY"=w1489, "VISA REFERENCE"=w1490) -> ("error out 15"=→"error out 37":errorcluster, "Read Buffer Array"=w1487:string[])  [unwired: 1 in]
                                }
                              }
                              n792 = Index Array(array=w1468, index=1) -> (element=w1482:string)
                              n793 = Equal?(x=w1478, y=0.0) -> (x = y?=w1474:bool)
                              n794 = Fract/Exp String To Number(string=w1482) -> (number=w1479:dbl)  [unwired: 3 in, 1 out]
                              n795 = Equal?(x=w1478, y=w1479) -> (x = y?=w1475:bool)
                              n796 = And(x=w1475, y=w1474) -> (x .and. y?=w1473:bool)
                              n797 = Equal?(x=w1479, y=w1481) -> (x = y?=w1472:bool)
                              n798 = Or(x=w1473, y=w1472) -> (x .or. y?=w1471:bool)
                              n799 = case shown="True" w1471 {
                                tunnel: [FALSE ("ABORT SWEEP") TRUE ("ABORT SWEEP")] -> w1480
                                tunnel: w1476 -> [_ w1495]
                                frame False {
                                }
                                frame True {
                                n800 = Add(x=1000.0, y=w1495) -> (x+y=w1494:dbl)
                                n801 = Wait (ms)(milliseconds to wait=w1494) -> ()  [unwired: 1 out]
                                }
                              }
                            }
                          }
                          frame True {
                            # "MIGHT HAVE TO SRQ HERE!"
                            n802 = while {
                              tunnel: w1501 -> [w1523]
                              tunnel: w1500 -> [w1522]
                              tunnel: w1499 -> [w1520]
                              tunnel: [w1519] -> w1498
                              tunnel: [w1508] -> w1497
                              stop <- w1509 stop-if-true
                              n803 = local read "ABORT SWEEP"() -> (w1510:bool)
                              n804 = call "VISAreadWrite.vi"("error in (no error)"=w1520, "GPIB INDEX Array"=i32[] [48], "GPIB ARRAY"=w1522, "VISA REFERENCE"=w1523) -> ("error out 15"=w1519:errorcluster, "Read Buffer Array"=w1518:string[])
                              n805 = Index Array(array=w1518, index=1) -> (element=w1515:string)
                              n806 = Decimal String To Number(string=w1515) -> (number=w1514:i32)  [unwired: 2 in, 1 out]
                              n807 = Quotient & Remainder(x=w1514, y=4) -> (x-y*floor(x/y)=w1512:i32)  [unwired: 1 out]
                              n808 = Wait (ms)(milliseconds to wait=u32 3000) -> ()  [unwired: 1 out]
                              n809 = Greater Or Equal?(x=w1512, y=2) -> (x >= y?=w1508:bool)
                              n810 = Or(x=w1510, y=w1508) -> (x .or. y?=w1509:bool)
                            }
                            n811 = case shown="True" w1497 {
                              tunnel: [w1525 w1535] -> _
                              tunnel: w1501 -> [_ w1534]
                              tunnel: w1500 -> [_ w1533]
                              tunnel: w1507 -> [_ w1532]
                              tunnel: w1506 -> [_ w1531]
                              tunnel: w1504 -> [_ w1530]
                              tunnel: w1503 -> [_ w1529]
                              tunnel: w1502 -> [_ w1528]
                              tunnel: w1498 -> [_ w1527]
                              frame False {
                                n812 = local read "ABORT SWEEP"() -> (w1524:bool)
                                n813 = Or(x=w1524, y=FALSE) -> (x .or. y?=w1525:bool)
                              }
                              frame True {
                                n814 = flat-sequence {
                                tunnel: [TRUE] -> w1535
                                tunnel: w1534 -> [w1548]
                                tunnel: w1533 -> [w1547]
                                tunnel: w1532 -> [w1561]
                                tunnel: w1531 -> [w1560]
                                tunnel: w1530 -> [w1558]
                                tunnel: w1529 -> [w1557]
                                tunnel: w1528 -> [w1539]
                                frame #0 {
                                n815 = Wait (ms)(milliseconds to wait=u32 2000) -> ()  [unwired: 1 out]
                                }
                                frame #1 {
                                n816 = call "VISAreadWrite.vi"("GPIB INDEX Array"=i32[] [38], "GPIB ARRAY"=w1547, "VISA REFERENCE"=w1548) -> ("error out 15"=w1543:errorcluster, "Read Buffer Array"=w1568:string[])  [unwired: 1 in]
                                n817 = local write "X Axis: LAST"(u16 66 ("milliseconds to wait")) -> ()
                                n818 = Index Array(array=w1568, index=3) -> (element=w1541:string)
                                n819 = Greater Or Equal?(x=w1539, y=i16 1) -> (x >= y?=w1537:bool)
                                n820 = case shown="True" w1537 {
                                tunnel: w1548 -> [_ w1577]
                                tunnel: w1547 -> [_ w1576]
                                tunnel: w1539 -> [_ w1575]
                                tunnel: "" -> [_ w1574]
                                tunnel: ["" w1573] -> w1544
                                tunnel: w1543 -> [_ w1572]
